vi "WebcamCheckTarget.vi"(8 "error in":errorcluster, 10 "TemplatePath":path=path "C:/Users/nalindquist/Desktop/WebcamTemplateGreen.png", 11 "ImageIn":T1) -> (0 "error out":errorcluster, 2 "MatchFound?":bool, 3 "Image Out":T1(plugin-control))   [LabVIEW 2015]
doc: "Processes the webcam image for a green rectangle. Returns true if at least one match was found."
uses:
  <vilib>/vision/Image Controls.llb/IMAQ Image.ctl
  <vilib>/vision/NI_Vision_Development_Module.lvlib
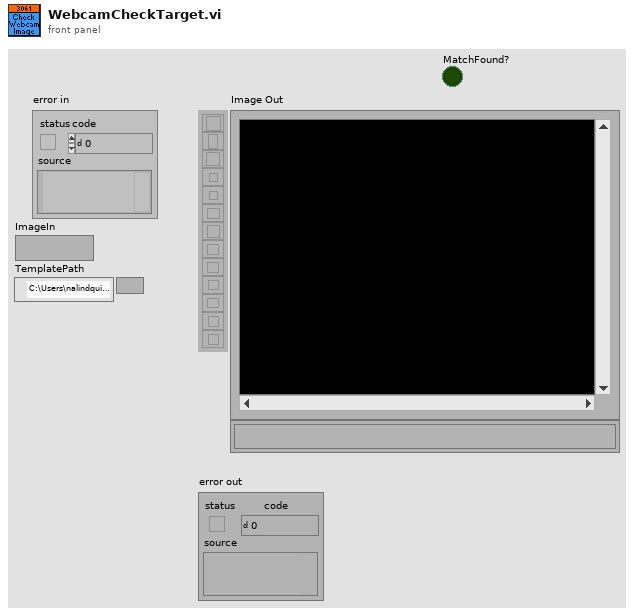
[diagram p1: front panel]
types:
  T1 = typedef "IMAQ Image.ctl" = refnum<image>
  T2 = typedef "Image Type" = u32
  T3 = cluster{"Global Rectangle":i32[], "Contours":cluster{"ID":enum32{"External", "Internal"}, "Type":u32, "Coordinates":i32[]}[]}
  T4 = cluster{"Position":cluster{"x":sgl, "y":sgl}, "Angle":sgl, "Scale":sgl, "Score":sgl, "Bounding Box":cluster{"x":sgl, "y":sgl}[]}[]
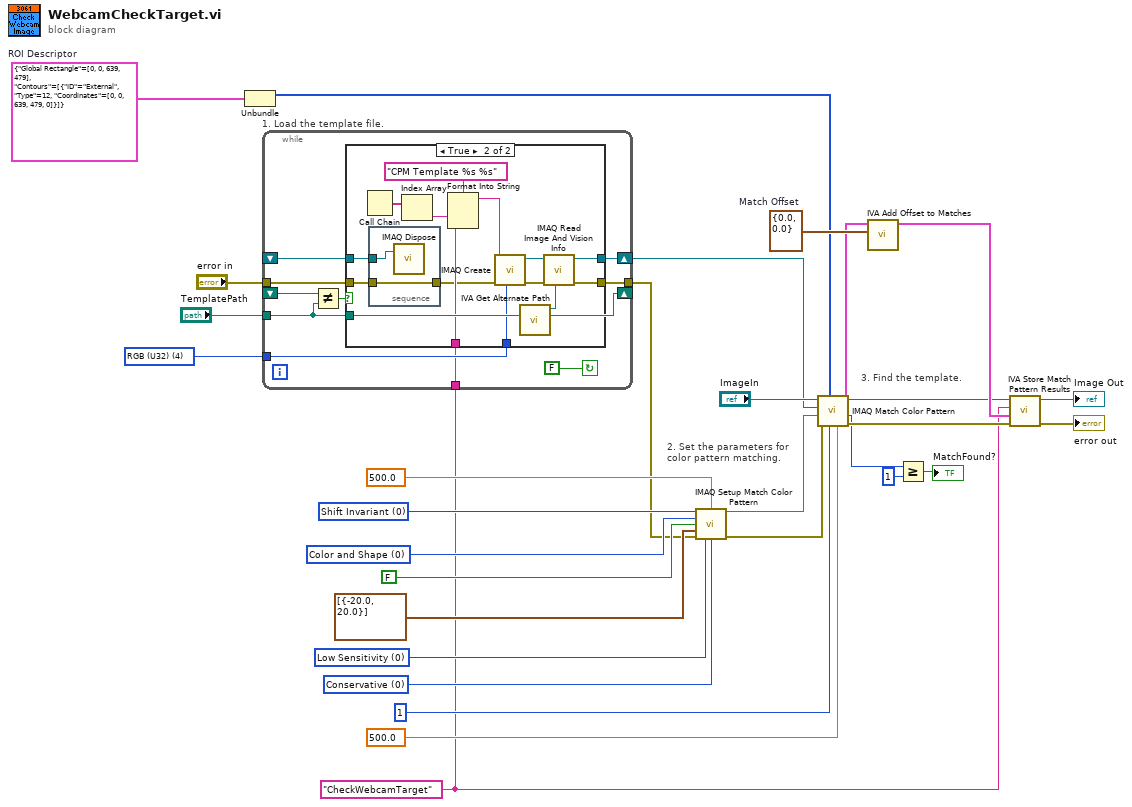
[diagram p0: block diagram]
diagram:
  w13 = "CheckWebcamTarget" ("Step Name")
  w20 = T2 4 items=["Grayscale (U8)", "Grayscale (I16)", "Grayscale (SGL)", "Complex (CSG)", "RGB (U32)", "HSL (U32)", "RGB (U64)"] ("Image Type")
  w18 = cluster{"X":sgl, "Y":sgl} {"X"=0.0, "Y"=0.0}  # Match Offset
  w23 = u32 0 items=["Conservative", "Balance", "Aggressive", "Very Aggressive"] ("Search Strategy")
  w24 = u32 0 items=["Low Sensitivity", "Medium Sensitivity", "High Sensitivity"] ("Color Sensitivity")
  w26 = u32 0 items=["Color and Shape", "Color", "Shape"] ("Match Feature Mode")
  w27 = u32 0 items=["Shift Invariant", "Rotation Invariant"] ("Match Mode")
  w17 = T3 {"Global Rectangle"=[0, 0, 639, 479], "Contours"=[{"ID"=enum."External", "Type"=12, "Coordinates"=[0, 0, 639, 479, 0]}]}  # ROI Descriptor
  # "2. Set the parameters for\ncolor pattern matching."
  # "3. Find the template."
  n1 = Unbundle(w17) -> ("Global Rectangle"=w7:i32[])  [unwired: 1 out]
  n2 = while "1. Load the template file." {
    shift-right: [w39] -> w6
    shift-left: _ -> [w38]
    tunnel: [w36] -> w5
    tunnel: "error in" -> [w35]
    tunnel: "TemplatePath" -> [w30]
    tunnel: w20 -> [w34]
    tunnel: w13 -> [w33]
    shift-right: [w30] -> _
    shift-left: _ -> [w32]
    stop <- FALSE continue-if-true
    n3 = Not Equal?(x=w32, y=w30) -> (x != y?=w31:bool)
    n4 = case shown="True" w31 {
      tunnel: [w41 w54] -> w39
      tunnel: w38 -> [w41 w46]
      tunnel: [w40 w51] -> w36
      tunnel: w35 -> [w40 w45]
      tunnel: w30 -> [_ w43]
      tunnel: w34 -> [_ w50]
      tunnel: w33 -> [_ w47]
      frame False {
      }
      frame True {
        n5 = Call Chain() -> (call chain=w49:string[])
        n6 = stacked-sequence {
          tunnel: w46 -> [w58]
          tunnel: w45 -> [w57]
          tunnel: [w57] -> w44
          frame #0 {
            n7 = call "IMAQ Dispose"("Image"=w58) -> ()  [unwired: 2 in, 4 out]
          }
        }
        n8 = Index Array(array=w49) -> (element=w48:string)  [unwired: 1 in]
        n9 = Format Into String(format string="CPM Template %s %s" ("Image Name"), w48, w47) -> (resulting string=w56:string)  [unwired: 2 in, 1 out]
        n10 = call "IMAQ Create"("Image Name"=w56, "Image Type"=w50, "error in (no error)"=w44) -> ("New Image"=w53:T1, "error out"=w52:errorcluster)  [unwired: 1 in, 1 out]
        n11 = call <vilib>:"IVA Get Alternate Path.vi"("Path In"=w43) -> ("Path Out"=w42:path)  [unwired: 10 out]
        n12 = call "IMAQ Read Image And Vision Info"("File Path"=w42, "error in (no error)"=w52, "Image"=w53) -> ("error out"=w51:errorcluster, "Image Out"=w54:T1)  [unwired: 1 in, 6 out]
      }
    }
  }
  n13 = call "IMAQ Setup Match Color Pattern"("Match Mode"=w27, "Color Score Weight"=sgl 500.0, "Match Feature Mode"=w26, "Subpixel Accuracy"=FALSE, "Rotation Angle Ranges (degrees)"=cluster{sgl, sgl}[] [{-20.0, 20.0}], "error in (no error)"=w5, "Color Sensitivity"=w24, "Search Strategy"=w23) -> ("Match Color Pattern Setup Data"=w10:string, "error out"=w9:errorcluster)  [unwired: 1 in, 5 out]
  n14 = call "IMAQ Match Color Pattern"("Minimum Match Score"=sgl 500.0, "Number of Matches Requested"=1, "Optional Rectangle"=w7, "error in (no error)"=w9, "Match Color Pattern Setup Data"=w10, "Template Image"=w6, "Image"="ImageIn") -> ("error out"=w15:errorcluster, "Number of Matches"=w3:i32, "Matches"=w8:T4)  [unwired: 2 out]
  n15 = call <vilib>:"IVA Add Offset to Matches.vi"("Match Offset"=w18, "Matches in"=w8) -> ("Matches out"=w16:T4)  [unwired: 9 out]
  n16 = Greater Or Equal?(x=w3, y=1) -> (x >= y?=→"MatchFound?":bool)
  n17 = call <vilib>:"IVA Store Match Pattern Results.vi"("error in (no error)"=w15, "Matches"=w16, "Step Name"=w13, "Image in"="ImageIn") -> ("error out"=→"error out":errorcluster, "Image dup"=→"Image Out":T1)  [unwired: 6 out]
